vi "Set System Image (Folder).vi"(4 "File and Directory Blacklist":string[](array[string]), 5 "Encryption Passphrase":string, 6 "Original System Only (F)":bool, 7 "Restart Automatically (T)":bool=TRUE, 8 "error in (no error)":errorcluster, 9 "Network Settings (preserve primary adapter, apply others)":T1=3 items=["reset all network adapters", "preserve primary, reset others", "preserve all network adapters", "preserve primary, apply others", "apply primary, reset others", "apply primary, preserve others", "apply all network adapters"], 10 "Source Folder":path, 11 "Session in":refnum<k21>) -> (0 "error out":errorcluster, 3 "Session out":refnum<k21>)   [LabVIEW 2020, in "nisyscfg.lvlib"]
doc: "Replaces the entire contents of the primary hard drive on a specified target system with an image folder created with the Create System Image VI."
uses:
  <vilib>/nisyscfg/nisyscfg.lvlib
  <vilib>/nisyscfg/Network Settings Image.ctl
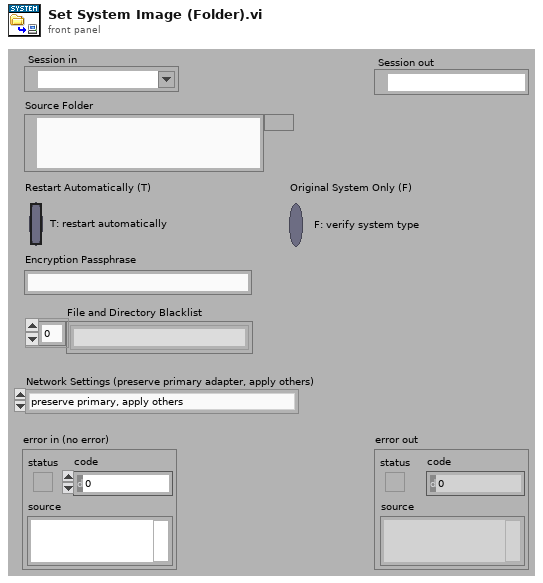
[diagram p1: front panel]
types:
  T1 = typedef "nisyscfg.lvlib/Network Settings Image.ctl" = u32
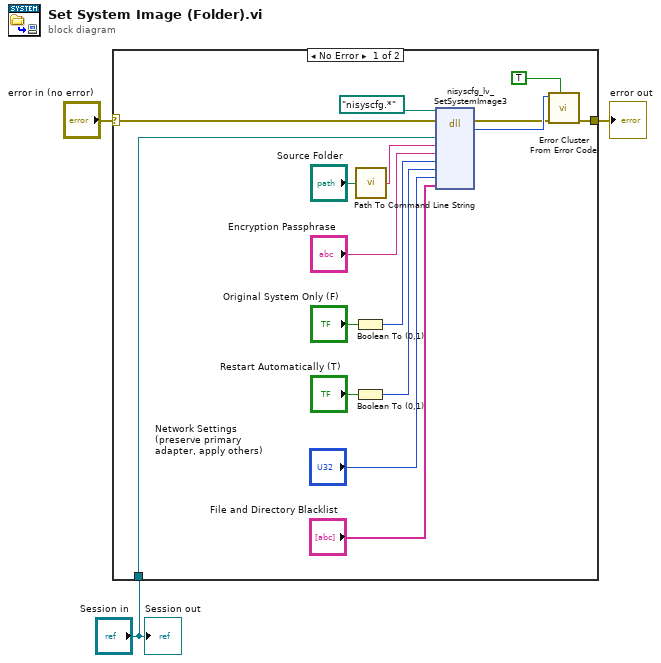
[diagram p0: block diagram]
diagram:
  n1 = case shown="No Error" "error in (no error)" {
    selector: "error in (no error)" -> [w14 w20]
    tunnel: [w19 w20] -> w3
    tunnel: "Session in" -> [w13 _]
    frame No Error {
      n2 = Boolean To (0,1)(Boolean="Original System Only (F)") -> (0, 1=w15:i16)
      n3 = Boolean To (0,1)(Boolean="Restart Automatically (T)") -> (0, 1=w9:i16)
      n4 = call <vilib>:"Path To Command Line String.vi"("path"="Source Folder") -> ("string"=w6:string)
      n5 = dll-call lib="nisyscfg.*" fn="nisyscfg_lv_SetSystemImage3" label="SetSystemImage"(path in=path "nisyscfg.*", error in=w14, "system"=w13, "localImagePath"=w6, "encryptionPassphrase"="Encryption Passphrase", "verifySystemID"=w15, "restartAutomatically"=w9, "networkSettings"="Network Settings (preserve primary adapter, apply others)", "blacklist"="File and Directory Blacklist") -> (error out=w17:errorcluster, "result"=w18:i32)  [unwired: 8 in, 1 out]
      n6 = call <vilib>:"Error Cluster From Error Code.vi"("show call chain? (False)"=TRUE, "error in (no error)"=w17, "error code (0)"=w18) -> ("error out"=w19:errorcluster)  [unwired: 6 in]
    }
    frame Error {
    }
  }
  "error out" <- w3
  "Session out" <- "Session in"
